vi "Set Idle.vi"(8 "error in (no error)":errorcluster, 10 "Idle":bool, 11 "Scorer in":refnum<class "Scorer.lvclass">) -> (0 "error out":errorcluster, 3 "Scorer out":refnum<class "Scorer.lvclass">)   [LabVIEW 2020, in "Summer of LabVIEW.lvlib" / "Scorer.lvclass"]
uses:
  Scorer.lvclass
  Scorer.lvclass/Scorer.ctl
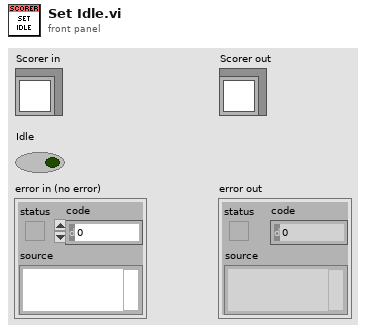
[diagram p1: front panel]
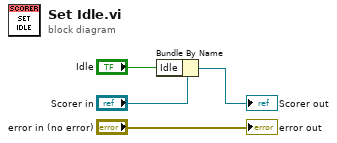
[diagram p0: block diagram]
diagram:
  n1 = Bundle By Name(cluster="Scorer in", "Idle"="Idle") -> (→"Scorer out":refnum<class "Scorer.lvclass">)
  "error out" <- "error in (no error)"
